vi "OAT Analog Tacho Process (N Tachos).vi"(0 "analog tacho signals":waveform(dbl)[](array[waveform]), 1 "missing pulses? (no:F)":bool[](array[boolean]), 2 "reset? (F)":bool, 5 "threshold (auto)":dbl[](array[numeric]) format="%.2f", 7 "pulse/revolution (1)":i32[](array[numeric]), 9 "hysteresis (0)":dbl[](array[numeric]) format="%.2f", 11 "error in (no error)":errorcluster, 12 "pulse width (2)":i32[](array[numeric]), 13 "slope (Rising)":u16[](array[ring]) items=["Rising", "Falling"]) -> (4 "speed profiles":T1[](array[typedef]) {"speed [RPM]" format="%.2f"; "time [s]" format="%.2f"}, 6 "actual threshold":dbl[](array[numeric]), 8 "speed position info":T2[](array[typedef]), 10 "no tacho?":bool[](array[boolean]), 15 "error out":errorcluster)   [LabVIEW 2017, in "SoundVib_TachProcess.lvlib"]
doc: "Locates tachometer pulse positions in analog tachometer signals using the number of generated pulses per revolution, the pulse width, and the arrival edge of the tachometer pulse. This VI also calculates the rotational speed of the device. Wire data to the <B>analog tacho signal</B> input to determine the polymorphic instance to use or manually select the instance."
uses:
  <vilib>/addons/Sound and Vibration/Order Analysis/Tach Process/SoundVib_TachProcess.lvlib
  <vilib>/addons/Sound and Vibration/Order Analysis/Misc/OAT Position Info.ctl
  <vilib>/addons/Sound and Vibration/Order Analysis/Tach Process/SubVIs/speed profile.ctl
  <vilib>/addons/_NISVFA/_Shared subVIs/Common/svc_Check for Waveform Parameter Continuity (no state).vi
  <vilib>/addons/_NISVFA/_Shared subVIs/Common/svc_Get SV Channel Info.vi
  <vilib>/addons/Sound and Vibration/Order Analysis/Tach Process/SubVIs/oa_Get Angular Speed (N Tach).vi
  <vilib>/addons/Sound and Vibration/Order Analysis/Tach Process/SubVIs/OAT Edge Detection (N Tach).vi
  <vilib>/Waveform/WDTOps.llb/WDT Waveform Duration DBL.vi
  <vilib>/addons/_NISVFA/_Shared subVIs/Common/svc_Engineering Units to Unit Label.vi
  <vilib>/addons/_NISVFA/_Shared subVIs/Common/svc_Unit Label to Engineering Units.vi
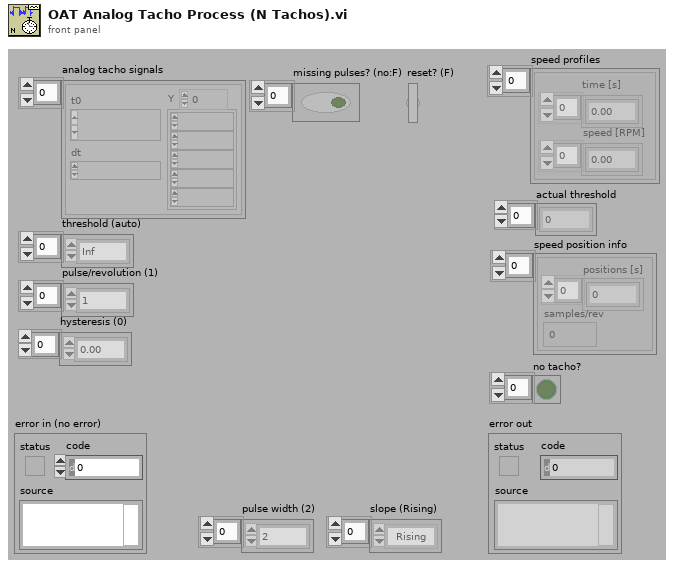
[diagram p1: front panel]
types:
  T1 = typedef "SoundVib_TachProcess.lvlib/speed profile.ctl" = cluster{"time [s]":dbl[], "speed [RPM]":dbl[]}
  T2 = typedef "OAT Position Info.ctl" = cluster{"positions [s]":dbl[], "samples/rev":dbl}
  T3 = cluster{"dt equal":bool, "array length equal":bool, "number channels change":bool}
  T4 = cluster{"dt":bool, "t0 continuity":bool, "array length":bool, "channel info":bool, "name":bool}
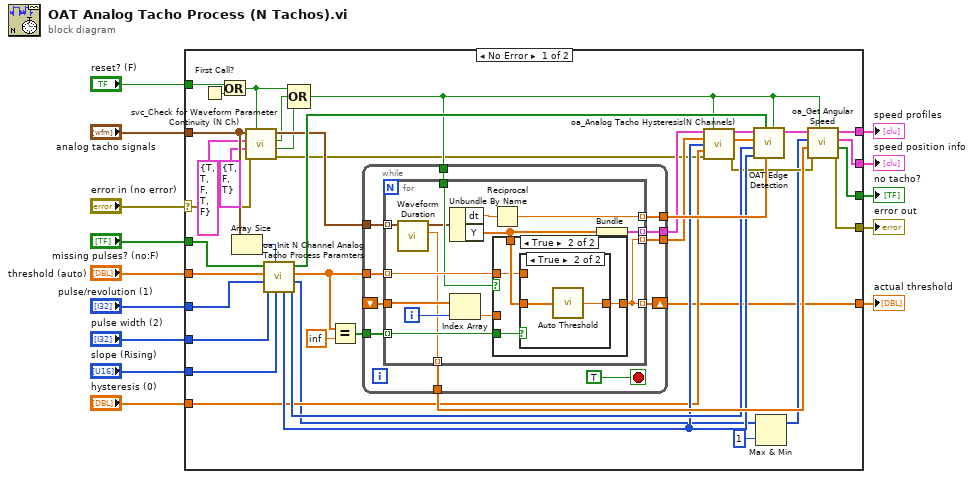
[diagram p0: block diagram]
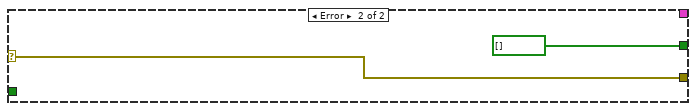
[diagram p4: hidden frame]
diagram:
  n1 = case shown="No Error" "error in (no error)" {
    selector: "error in (no error)" -> [w20 w89]
    tunnel: "threshold (auto)" -> [w45 _]
    tunnel: [w52 _] -> w13
    tunnel: [w53 w89] -> w12
    tunnel: [w51 bool[] []] -> w11
    tunnel: [w54 _] -> w10
    tunnel: "analog tacho signals" -> [w26 _]
    tunnel: "missing pulses? (no:F)" -> [w41 _]
    tunnel: "pulse/revolution (1)" -> [w40 _]
    tunnel: "pulse width (2)" -> [w39 _]
    tunnel: "slope (Rising)" -> [w38 _]
    tunnel: "hysteresis (0)" -> [w30 _]
    tunnel: "reset? (F)" -> [w18 _]
    tunnel: [w17 _] -> w1
    frame No Error {
      n2 = First Call?() -> (First Call?: T/F=w37:bool)
      n3 = Or(x=w18, y=w37) -> (x .or. y?=w24:bool)
      n4 = Array Size(array=w26) -> (size(s)=w46:i32)
      n5 = call <vilib>:"svc_Check for Waveform Parameter Continuity (N Ch).vi"("restart averaging (F)"=w24, "error in (no error)"=w20, "checks for multichannel parameters"=T3 {"dt equal"=TRUE, "array length equal"=FALSE, "number channels change"=TRUE}, "checks for channel parameter change"=T4 {"dt"=TRUE, "t0 continuity"=TRUE, "array length"=FALSE, "channel info"=TRUE, "name"=FALSE}, "scaled signal(s)"=w26) -> ("error out"=w19:errorcluster, "multichannel parameter changed"=w22:bool, "waveform parameter changed"=w23:bool, "dup scaled signal(s)"=w25:waveform(dbl)[])  [unwired: 3 out]
      n6 = call <vilib>:"oa_Init N Channel Analog Tacho Process Paramters.vi"("slope (Rising)"=w38, "channel number"=w46, "pulse width (2)"=w39, "pulse/revolution (1)"=w40, "threshold (auto)"=w45, "missing pulses? (no:F)"=w41) -> ("pulse width out"=w44:i32[], "pulse/revolution out"=w29:i32[], "threshold out"=w43:dbl[], "missing pulses? out"=w42:bool[], "slope out"=w33:u16[])  [unwired: 1 in]
      n7 = Compound Arithmetic op=OR(w24, w23, w22) -> (w21:bool)
      n8 = Equal?(x=w43, y=inf) -> (x = y?=w49:bool[])
      n9 = while {
        tunnel: w25 -> [w65]
        tunnel: w21 -> [w64]
        tunnel: w49 -> [w63]
        tunnel: w43 -> [w62]
        tunnel: [w61] -> w34
        tunnel: [w60] -> w35
        tunnel: [w59] -> w48
        shift-right: [w57] -> w17
        shift-left: _ -> [w58]
        tunnel: [w55] -> w47
        stop <- TRUE stop-if-true
        n10 = for {
          tunnel: [w71] -> w60 mode=indexing
          tunnel: [w75] -> w61 mode=indexing
          tunnel: w63 -> [w78] mode=indexing
          tunnel: w62 -> [w77] mode=indexing
          tunnel: w64 -> [w76]
          tunnel: w65 -> [w68] mode=indexing
          tunnel: [w75] -> w57 mode=indexing
          tunnel: w58 -> [w74]
          tunnel: [w69] -> w59 mode=indexing
          tunnel: [w66] -> w55 mode=indexing
          i -> [w73]
          n11 = call-poly <vilib>:"Waveform Duration.vi"("waveform in"=w68) -> ("duration"=w66:dbl, "waveform out"=w67:waveform(dbl))  [unwired: 8 in, 1 out]
          n12 = Unbundle By Name(w67) -> ("dt"=w70:dbl, "Y"=w79:dbl[])
          n13 = Index Array(array=w74, index=w73) -> (element=w72:dbl)
          n14 = Reciprocal(x=w70) -> (1/x=w69:dbl)
          n15 = case shown="True" w76 {
            tunnel: w79 -> [_ w84]
            tunnel: [w80 w83] -> w75
            tunnel: w72 -> [w80 _]
            tunnel: w77 -> [_ w82]
            tunnel: w78 -> [_ w81]
            frame False {
            }
            frame True {
              n16 = case shown="True" w81 {
                tunnel: w84 -> [_ w87]
                tunnel: [w85 w86] -> w83
                tunnel: w82 -> [w85 _]
                frame False {
                }
                frame True {
                  n17 = call <vilib>:"Auto Threshold.vi"("x[n]"=w87) -> ("threshold"=w86:dbl)
                }
              }
            }
          }
          n18 = Bundle("Y"=w79) -> (w71:cluster{"Y":dbl[]})  [unwired: 1 in]
        }
      }
      n19 = call <vilib>:"oa_Analog Tacho Hysteresis(N Channels).vi"("input signal"=w35, "reset? (T)"=w21, "threshold (auto)"=w34, "slope (Rising)"=w33, "hysteresis(0)"=w30, "error in (no error)"=w19) -> ("output signal"=w31:cluster{"Signal":dbl[]}[], "error out"=w32:errorcluster)  [unwired: 8 in]
      n20 = call-poly <vilib>:"OAT Edge Detection.vi"("reset? (True)"=w21, "sampling frequency [Hz]"=w48, "missing pulses? (no:F)"=w42, "slope (Rising)"=w33, "pulse width (2)"=w44, "threshold (0.0)"=w34, "x(n)"=w31) -> ("pulse position [s]"=w36:cluster{dbl[]}[])  [unwired: 3 in, 1 out]
      n21 = Max & Min(x=w29, y=1) -> (max(x,y)=w28:i32[])  [unwired: 1 out]
      n22 = call-poly <vilib>:"oa_Get Angular Speed.vi"("reset? (True)"=w21, "error in (no error)"=w32, "durations"=w47, "pulse/revolution (1)"=w28, "pulse position [s]"=w36) -> ("error out"=w53:errorcluster, "No Tach? (False)"=w51:bool[], "speed position info"=w52:T2[], "speed profile"=w54:T1[])  [unwired: 3 in]
    }
    frame Error {
    }
  }
  "error out" <- w12
  "speed position info" <- w13
  "no tacho?" <- w11
  "speed profiles" <- w10
  "actual threshold" <- w1
